vi "SS_SORT_DATA.vi"(6 "Main Cluster IN":T1, 8 "Error In":errorcluster, 9 "Drop1 Data IN":fxp[][](array[numeric]), 10 "Drop0 Data IN":fxp[][](array[numeric]), 11 "Info In":string="\nWaiting for TimerScope Trigger\n- IN: SS TimerScope Trigger\n- OUT: SET SS ThermoRec Received Trigger\nPulse Number is 231123\nPulse Type is 4\n\nDuration (s) is  2.000000\nDelay (s)  is  1.000000\nScan Period (ms) is  15\nNumber of Samples is  134\n\nDelay Started\nDelay Complete\nExternal Measurement of Delay (s): 1.000000\nACQUIRING DATA") -> (0 "Error Out":errorcluster, 3 "Info Out":string="\nWaiting for TimerScope Trigger\n- IN: SS TimerScope Trigger\n- OUT: SET SS ThermoRec Received Trigger\nPulse Number is 231123\nPulse Type is 4\n\nDuration (s) is  2.000000\nDelay (s)  is  1.000000\nScan Period (ms) is  15\nNumber of Samples is  134\n\nDelay Started\nDelay Complete\nExternal Measurement of Delay (s): 1.000000\nACQUIRING DATA", 4 "Main Cluster OUT":T1)   [LabVIEW 2016]
uses:
  Control/Control_Main.ctl
  Control/Control_ModuleArray.ctl
panel:
  out "Drop1 Calibrated Thermocouple Data Out":dbl[][](array[numeric])
  out "Drop0 Calibrated Thermocouple Data Out":dbl[][](array[numeric])
  in  "Tab Control":enum32{"IN", "OUT", "SubVI Info", "FPGA"}(tab)
  out "Input Array Size":dbl[](array[numeric])
  out "Debug String":string
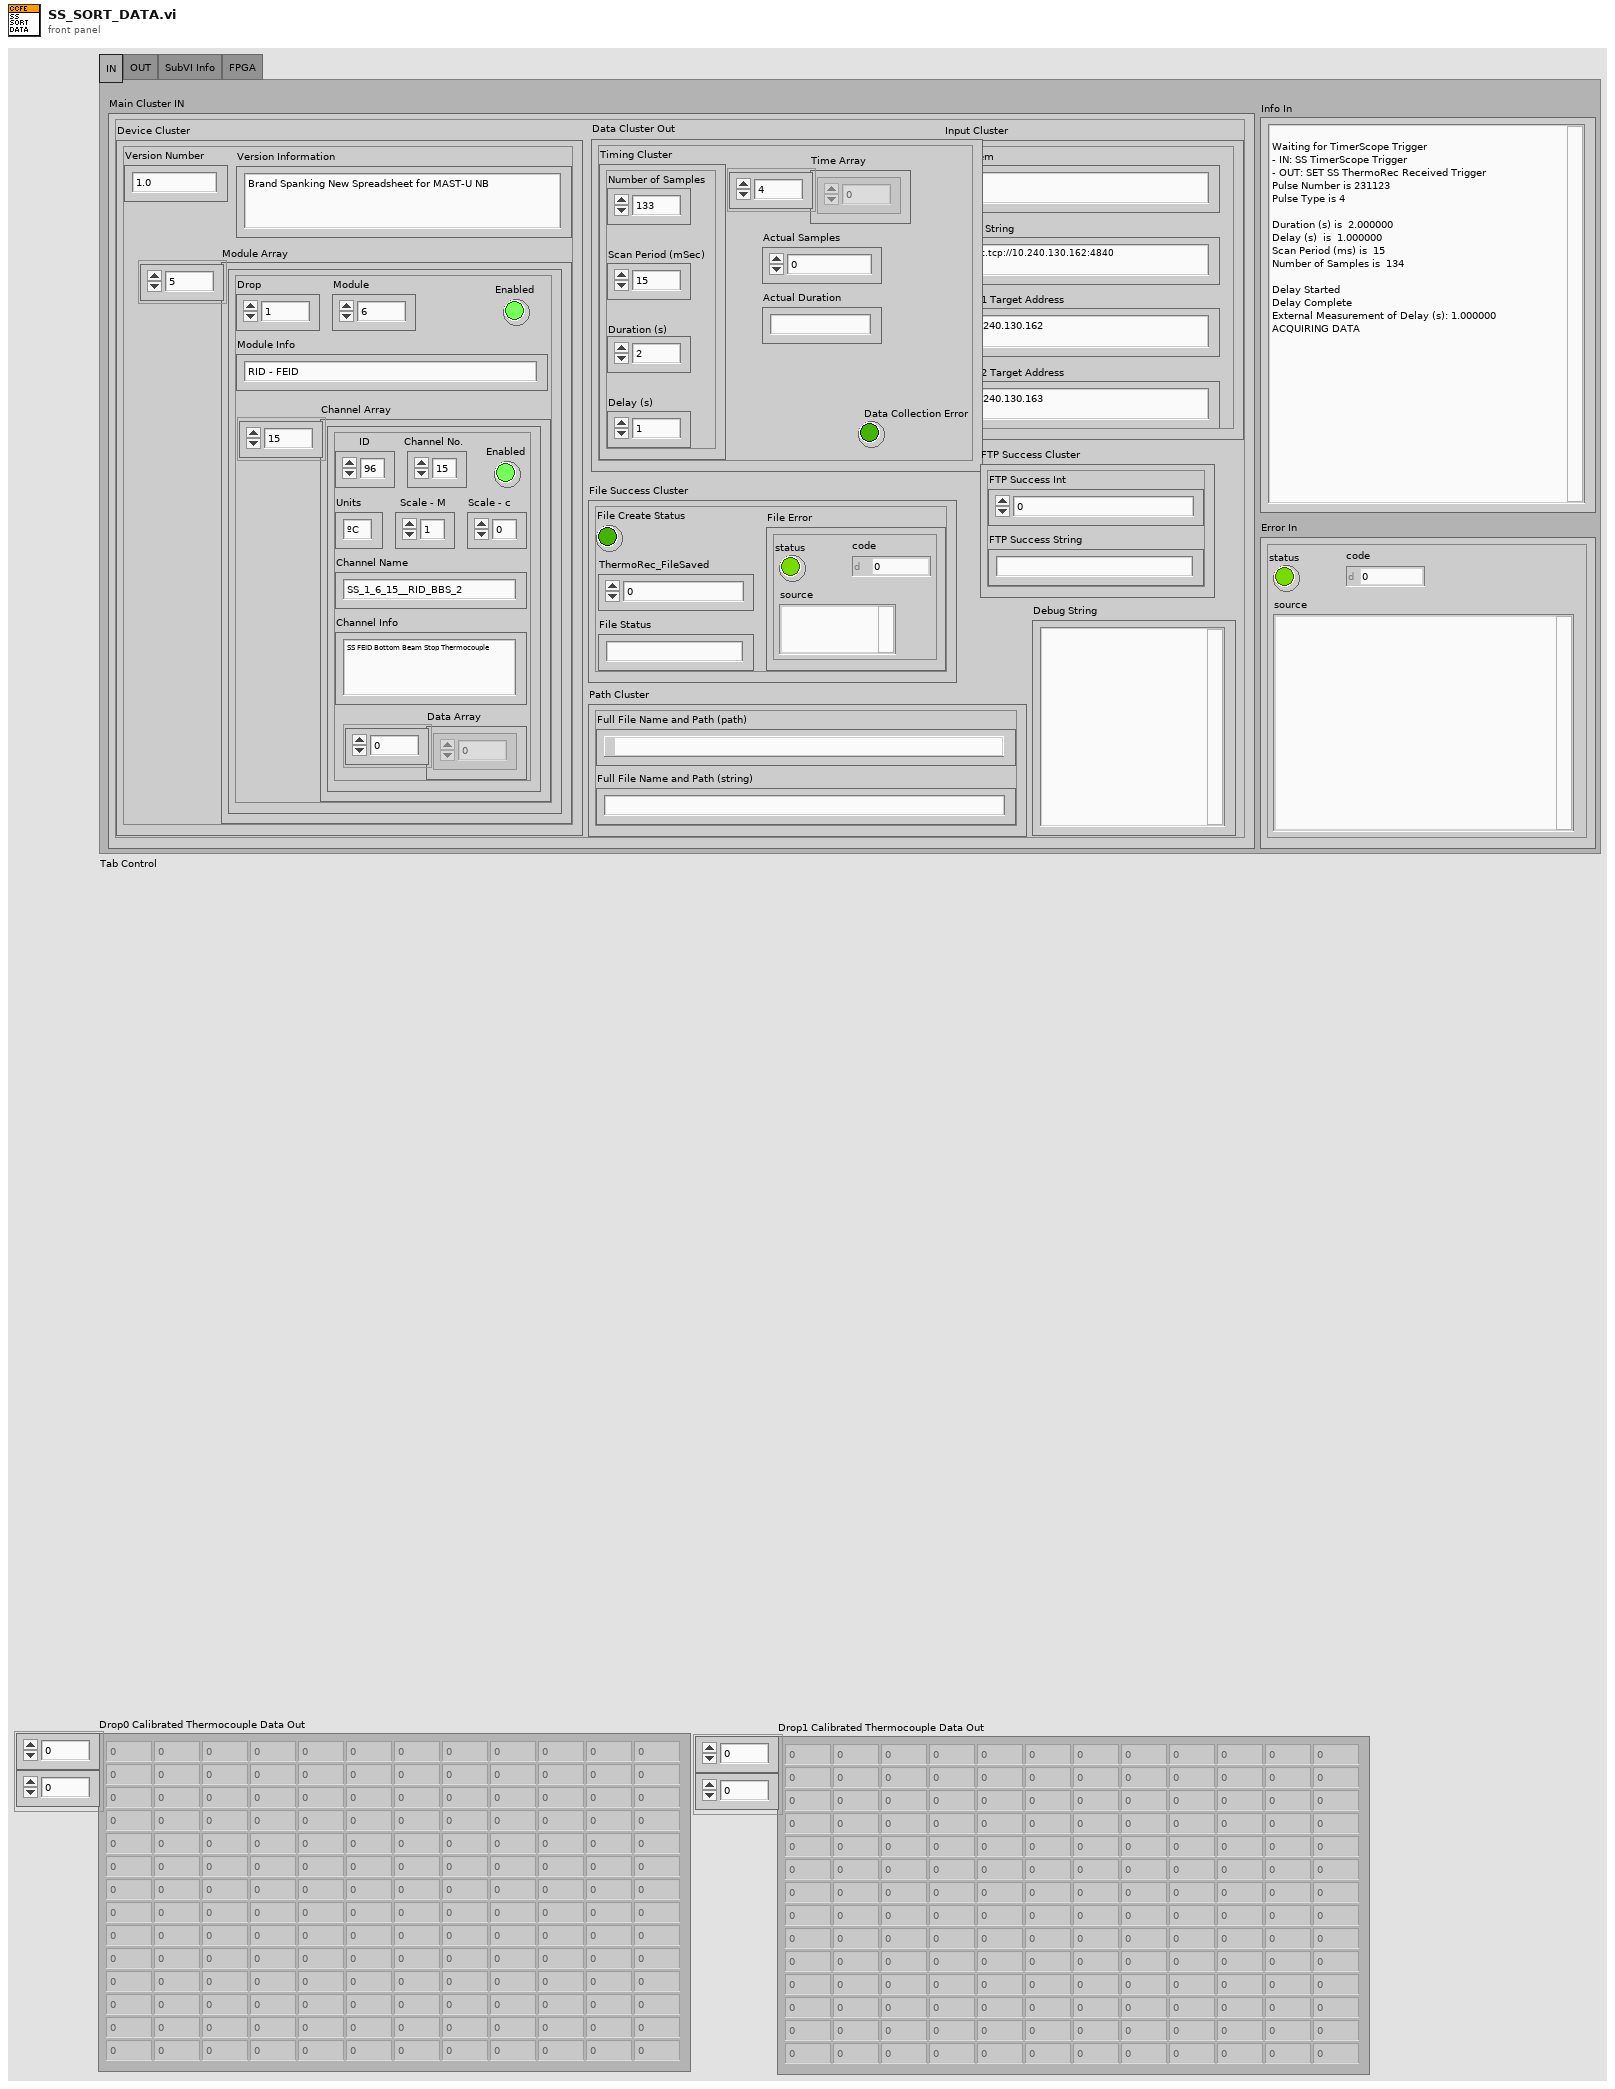
[diagram p1: front panel]
types:
  T1 = typedef "Control_Main.ctl" = cluster{"Device Cluster":cluster{"Module Array":T2, "Version Number":string, "Version Information":string}, "Input Cluster":cluster{"Input String":string, "Drop1 Target Address":string, "Drop2 Target Address":string, "System":string}, "Data Cluster Out":cluster{"Timing Cluster":cluster{"Number of Samples":i32, "Scan Period (mSec)":u32, "Duration (s)":dbl, "Delay (s)":dbl}, "Time Array":dbl[], "Actual Samples":i32, "Actual Duration":string, "Data Collection Error":bool}, "Path Cluster":cluster{"Full File Name and Path (path)":path, "Full File Name and Path (string)":string}, "File Success Cluster":cluster{"ThermoRec_FileSaved":i32, "File Create Status":bool, "File Error":errorcluster, "File Status":string}, "FTP Success Cluster":cluster{"FTP Success Int":i32, "FTP Success String":string}, "Debug String":string}
  T2 = typedef "Control_ModuleArray.ctl" = cluster{"Drop":i32, "Module":i32, "Module Info":string, "Enabled":bool, "Channel Array":cluster{"ID":i32, "Channel No.":i32, "Enabled":bool, "Channel Name":string, "Channel Info":string, "Units":string, "Scale - M":dbl, "Scale - c":dbl, "Data Array":dbl[]}[]}[]
  T3 = cluster{"ID":i32, "Channel No.":i32, "Enabled":bool, "Channel Name":string, "Channel Info":string, "Units":string, "Scale - M":dbl, "Scale - c":dbl, "Data Array":dbl[]}[]
  T4 = cluster{"ID":i32, "Channel No.":i32, "Enabled":bool, "Channel Name":string, "Channel Info":string, "Units":string, "Scale - M":dbl, "Scale - c":dbl, "Data Array":dbl[]}
  T5 = cluster{"Drop":i32, "Module":i32, "Module Info":string, "Enabled":bool, "Channel Array":cluster{"ID":i32, "Channel No.":i32, "Enabled":bool, "Channel Name":string, "Channel Info":string, "Units":string, "Scale - M":dbl, "Scale - c":dbl, "Data Array":dbl[]}[]}
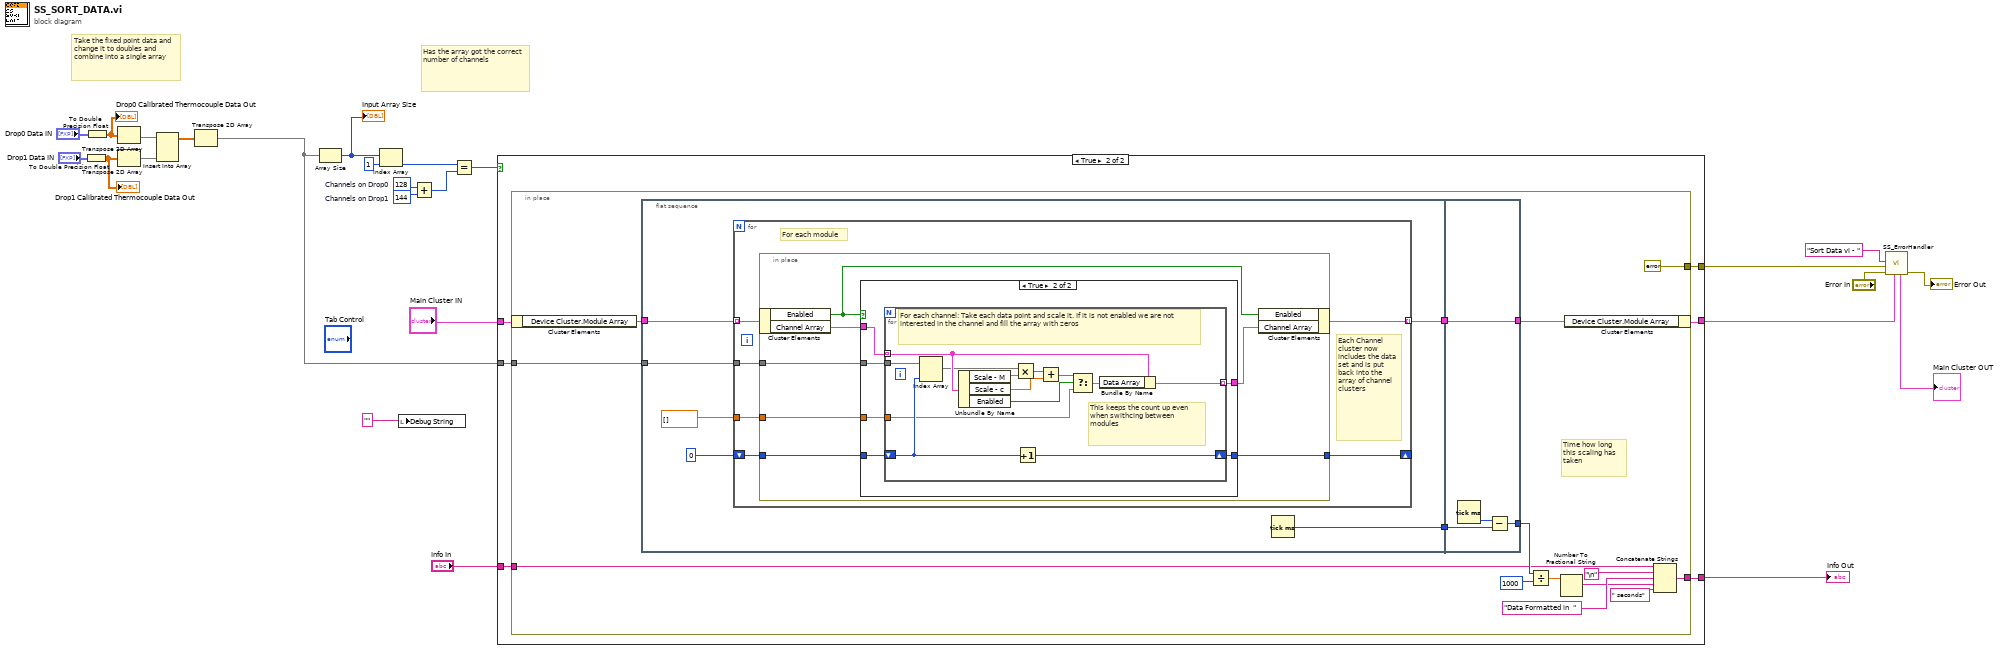
[diagram p0: block diagram]
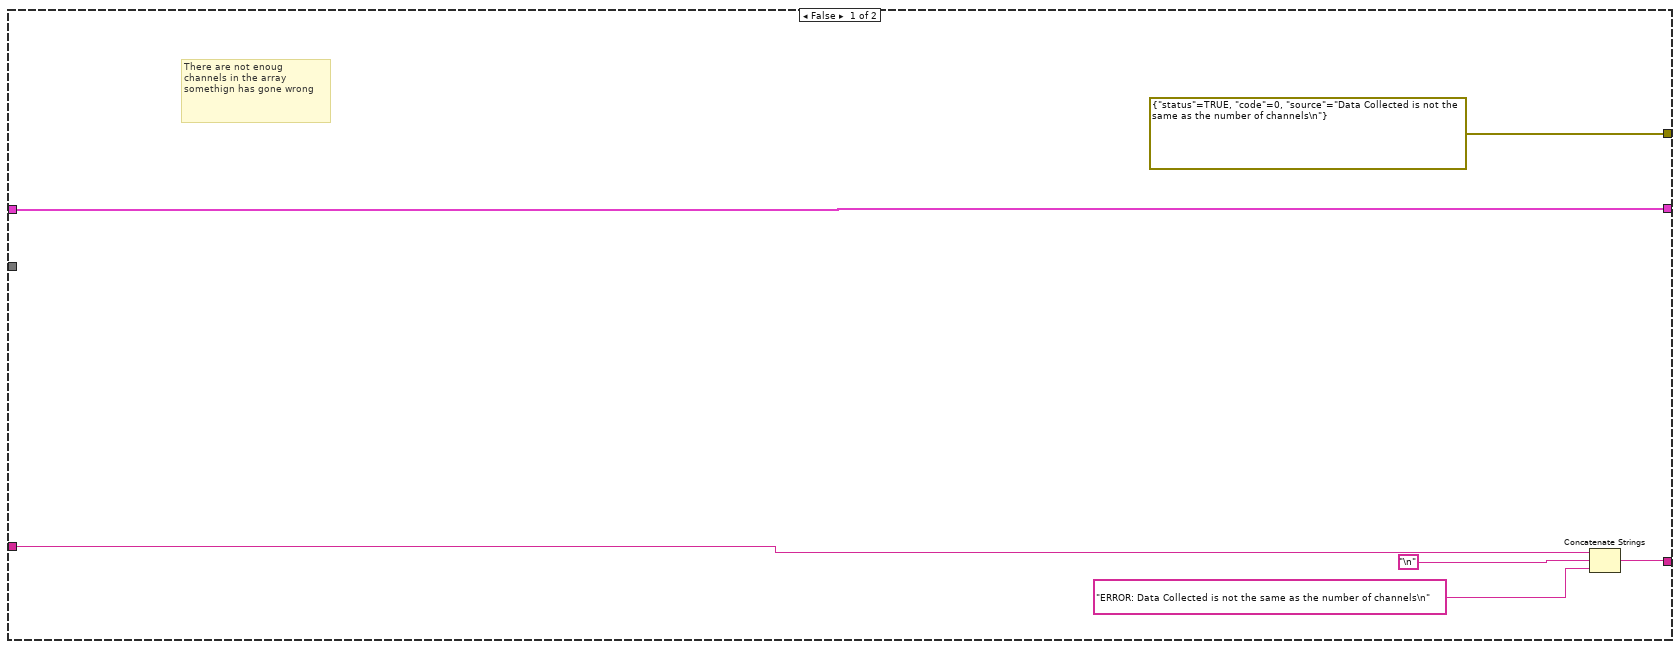
[diagram p2: hidden frame]
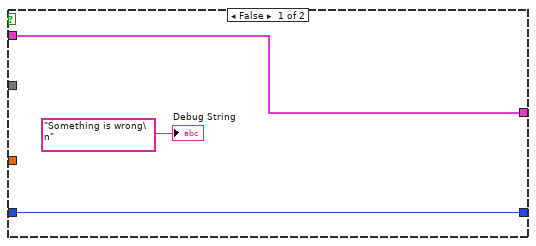
[diagram p3: hidden frame]
diagram:
  w12 = 144  # Channels on Drop1
  w13 = 128  # Channels on Drop0
  # "Has the array got the correct number of channels"
  # "Take the fixed point data and change it to doubles and combine into a single array"
  n1 = To Double Precision Float(number="Drop1 Data IN") -> (double precision float=w1:dbl[][])
  "Drop1 Calibrated Thermocouple Data Out" <- w1
  n2 = To Double Precision Float(number="Drop0 Data IN") -> (double precision float=w2:dbl[][])
  "Drop0 Calibrated Thermocouple Data Out" <- w2
  n3 = Transpose 2D Array(2D array=w2) -> (transposed array=w10:dbl[][])
  n4 = Transpose 2D Array(2D array=w1) -> (transposed array=w9:dbl[][])
  n5 = Insert Into Array(array=w10, new element=w9) -> (w7:dbl[][])  [unwired: 2 in]
  n6 = Transpose 2D Array(2D array=w7) -> (transposed array=w8:dbl[][])
  n7 = Array Size(array=w8) -> (size(s)=w25:i32[])
  "Input Array Size" <- w25
  n8 = Index Array(array=w25, index=1) -> (element=w23:i32)
  n9 = local write "Debug String"("") -> ()
  n10 = Add(x=w13, y=w12) -> (x+y=w11:i32)
  n11 = Equal?(x=w23, y=w11) -> (x = y?=w22:bool)
  n12 = case shown="True" w22 {
    tunnel: w8 -> [_ w32]
    tunnel: "Main Cluster IN" -> [w31 w34]
    tunnel: [w31 w35] -> w15
    tunnel: "Info In" -> [w27 w33]
    tunnel: [w28 w37] -> w20
    tunnel: [errorcluster {"status"=TRUE, "code"=0, "source"="Data Collected is not the same as the number of channels\n"} ("error constant") w36] -> w16
    frame False {
      # "There are not enoug channels in the array somethign has gone wrong"
      n13 = Concatenate Strings(w27, "\n", "ERROR: Data Collected is not the same as the number of channels\n") -> (w28:string)
    }
    frame True {
      n14 = in-place {
        in-place-border: [w41] -> w37
        in-place-border: [errorcluster {"status"=FALSE, "code"=0, "source"=""} ("error constant")] -> w36
        in-place-border: w33 -> [w39]
        in-place-border: w32 -> [w38]
        # "Time how long this scaling has taken"
        n15 = in-place-cluster #1(w34) -> ("Device Cluster.Module Array"=w43:T2)
        n16 = flat-sequence {
          tunnel: w43 -> [w54]
          tunnel: [w57] -> w52
          tunnel: [w56] -> w51
          tunnel: w38 -> [w53]
          tunnel: [w97] -> w42
          tunnel: w52 -> [w97]
          tunnel: w51 -> [w96]
          tunnel: [w94] -> w50
          frame #0 {
            n17 = for {
              tunnel: w54 -> [w61] mode=indexing
              tunnel: dbl[] [] -> [w64]
              tunnel: [w60] -> w57 mode=indexing
              shift-right: [w62] -> _
              shift-left: 0 -> [w63]
              tunnel: w53 -> [w59]
              # "Each Channel cluster now includes the data set and is put back into the array of channel clusters"
              # "For each module"
              n18 = in-place {
                in-place-border: w64 -> [w71]
                in-place-border: w63 -> [w70]
                in-place-border: [w69] -> w62
                in-place-border: w59 -> [w66]
                n19 = in-place-cluster #2(w61) -> ("Enabled"=w65:bool, "Channel Array"=w68:T3)
                n20 = case shown="True" w65 {
                  tunnel: w68 -> [w74 w79]
                  tunnel: w71 -> [_ w80]
                  tunnel: [w74 w78] -> w67
                  tunnel: w70 -> [w72 w77]
                  tunnel: [w72 w76] -> w69
                  tunnel: w66 -> [_ w75]
                  frame False {
                    "Debug String" <- "Something is wrong\n"
                  }
                  frame True {
                    n21 = for {
                      tunnel: w79 -> [w92] mode=indexing
                      tunnel: w80 -> [w83]
                      tunnel: [w93] -> w78 mode=indexing
                      shift-right: [w81] -> w76
                      shift-left: w77 -> [w87]
                      tunnel: w75 -> [w85]
                      # "This keeps the count up even when swithcing between modules"
                      # "For each channel: Take each data point and scale it. If it is not enabled we are not interested in the channel and fill the array with zeros"
                      n22 = Index Array(array=w85, index (col)=w87) -> (element=w82:dbl[])  [unwired: 1 in]
                      n23 = Unbundle By Name(w92) -> ("Scale - M"=w91:dbl, "Scale - c"=w89:dbl, "Enabled"=w86:bool)
                      n24 = Multiply(x=w82, y=w91) -> (x*y=w90:dbl[])
                      n25 = Increment(x=w87) -> (x+1=w81:i32)
                      n26 = Add(x=w90, y=w89) -> (x+y=w88:dbl[])
                      n27 = Select(t=w88, s=w86, f=w83) -> (s? t:f=w84:dbl[])
                      n28 = Bundle By Name(cluster=w92, "Data Array"=w84) -> (w93:T4)
                    }
                  }
                }
                n29 = in-place-cluster #2("Enabled"=w65, "Channel Array"=w67) -> (w60:T5)
              }
            }
            n30 = Tick Count (ms)() -> (millisecond timer value=w56:u32)
          }
          frame #1 {
            n31 = Tick Count (ms)() -> (millisecond timer value=w95:u32)
            n32 = Subtract(x=w95, y=w96) -> (x-y=w94:u32)
          }
        }
        n33 = Divide(x=w50, y=u32 1000) -> (x/y=w49:dbl)
        n34 = Number To Fractional String(number=w49) -> (F-format string=w44:string)  [unwired: 3 in]
        n35 = in-place-cluster #1("Device Cluster.Module Array"=w42) -> (w35:T1)
        n36 = Concatenate Strings(w39, "\n", "Data Formatted in  ", w44, " seconds") -> (w41:string)
      }
    }
  }
  "Info Out" <- w20
  n37 = call "SS_ErrorHandler.vi"("Main Cluster IN"=w15, "Error In"="Error In", "SubVI Error"=w16, "SubVI Name"="Sort Data vi - ") -> ("Error Out"=→"Error Out":errorcluster, "Main Cluster OUT"=→"Main Cluster OUT":T1)  [unwired: 5 in, 1 out]
